vi "DSF.Engine.Plugin.Rx.Transfer Group.Move Data.vi"(8 "error in (no error)":errorcluster, 10 "Transfer Group in":refnum<class "DSF.Engine.Transfer Group.lvclass">, 11 "Plugin in":refnum<class "DSF.Engine.Plugin.lvclass">) -> (0 "error out":errorcluster, 2 "Transfer Group out":refnum<class "DSF.Engine.Transfer Group.lvclass">, 3 "Plugin out":refnum<class "DSF.Engine.Plugin.lvclass">)   [LabVIEW 2017, in "Data Sharing Framework Engine.lvlib" / "DSF.Engine.Plugin.lvclass"]
uses:
  DSF.Engine.Plugin.lvclass
  Transfer/DSF.Engine.Transfer Group.lvclass
  Transfer/DSF.Engine.Transfer Group.lvclass/DSF.Engine.Transfer Group.ctl
  Transfer/DSF.Engine.Transfer.lvclass/DSF.Engine.Transfer.ctl
  <vilib>/National Instruments/Memory Manager/Classes/Pointer/Memory.Pointer.lvclass/Memory.Pointer.ctl
  Transfer/DSF.Engine.Transfer Group.Get Transfers.vi
  Transfer/DSF.Engine.Transfer.Get Inline Buffer.vi
  Transfer/DSF.Engine.Transfer.Get Intermediate Buffer.vi
  <vilib>/National Instruments/Memory Manager/Classes/Pointer/Memory.Pointer.Copy All.vi
  <vilib>/National Instruments/Memory Manager/Classes/Pointer/Memory.Pointer.Get Size.vi
  <vilib>/National Instruments/Memory Manager/Classes/Pointer/Memory.Pointer.Copy.vi
  <vilib>/National Instruments/Memory Manager/Classes/Pointer/Memory.Pointer.Copy.No Check.vi
  <vilib>/National Instruments/Memory Manager/Classes/Pointer/Memory.Pointer.Parameter Check.Subset.vi
  <vilib>/National Instruments/Memory Manager/Classes/Pointer/Memory.Pointer.Parameter Check.Null Pointer.vi
  <vilib>/National Instruments/Memory Manager/Classes/Pointer/Memory.Pointer.Get Address.vi
  <vilib>/National Instruments/Memory Manager/Classes/Pointer/Memory.Pointer.Errors.vi
  <vilib>/National Instruments/Memory Manager/Classes/Pointer/Memory.Pointer.Errors.Out of Bounds.vi
  <vilib>/National Instruments/Memory Manager/Classes/Pointer/Memory.Pointer.Errors.Null Pointer.vi
  <vilib>/NI/Static Error Handling/VIs/Static Error Handling.Source Buffer.Write.String.vi
  <vilib>/National Instruments/Memory Manager/Classes/Pointer/Memory.Pointer.Errors.Write Pointer Size.vi
  <vilib>/National Instruments/Memory Manager/Classes/Pointer/Memory.Pointer.Errors.Create Error.vi
  <vilib>/NI/Static Error Handling/VIs/Static Error Handling.Source Buffer.Write.Numeric.Scalar.Base10.vi
  <vilib>/NI/Static Error Handling/VIs/Static Error Handling.Source Buffer.Write.Numeric.Scalar.Base10 (U64).vi
  <vilib>/NI/Static Error Handling/VIs/Static Error Handling.Error Cluster Constant.vi
  <vilib>/NI/Static Error Handling/VIs/Static Error Handling.Error Cluster Constant (512B).vi
  <vilib>/NI/Static Error Handling/VIs/Static Error Handling.Parameters.Status.Set.vi
  <vilib>/NI/Static Error Handling/VIs/Static Error Handling.Parameters.Code.Set.vi
  <vilib>/NI/Static Error Handling/VIs/Static Error Handling.Parameters.VI Source.Set.vi
  <vilib>/National Instruments/Memory Manager/Constants/Memory.Constants.vi
  <vilib>/National Instruments/Memory Manager/Constants/Memory.Constants.Library Name.vi
  <vilib>/National Instruments/Memory Manager/Classes/Pointer/Memory.Pointer.Errors.Get Info.vi
  Source/Data Sharing Framework Core/Engine/Memory/Double Pointer/Double Pointer.lvclass
  C:/Program Files (x86)/National Instruments/LabVIEW 2017/vi.lib/National Instruments/Memory Manager/Classes/Pointer/Memory.Pointer.lvclass
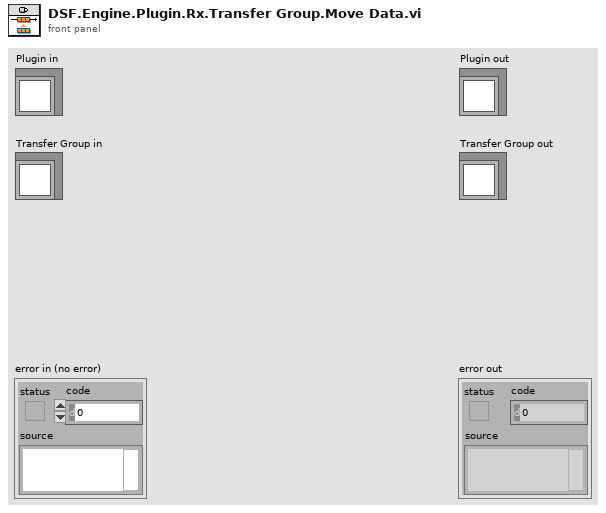
[diagram p1: front panel]
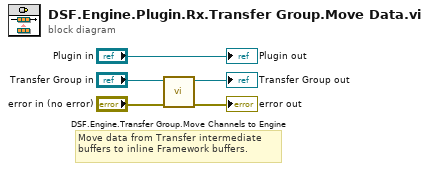
[diagram p0: block diagram]
diagram:
  # "Move data from Transfer intermediate buffers to inline Framework buffers."
  n1 = call "DSF.Engine.Transfer Group.Move Channels to Engine.vi"("error in (no error)"="error in (no error)", "Transfer Group in"="Transfer Group in") -> ("error out"=→"error out":errorcluster, "Transfer Group out"=→"Transfer Group out":refnum<class "DSF.Engine.Transfer Group.lvclass">)  [unwired: 8 in]
  "Plugin out" <- "Plugin in"
